vi "Init log file.vi"(8 "error in (no error)":errorcluster, 11 "Channel in":refnum<class "Channel.lvclass">) -> (0 "error out":errorcluster, 3 "Channel out":refnum<class "Channel.lvclass">)   [LabVIEW 2018, in "Channel.lvclass"]
uses:
  Channel.lvclass
  Error log/Error log.lvclass
  C:/Users/Denis/Desktop/S4ACS/SPARC4_ACS/Log File/Log File.lvclass
  Keywords Log File/Keywords Log File.lvclass
  Channel.lvclass/Channel.ctl
  Log File/Log File.lvclass/Log File.ctl
  Log File/Log File.lvclass
panel:
  in  "Keywords Log File.lvclass":refnum<class "Keywords Log File.lvclass">
  in  "Error log.lvclass":refnum<class "Error log.lvclass">
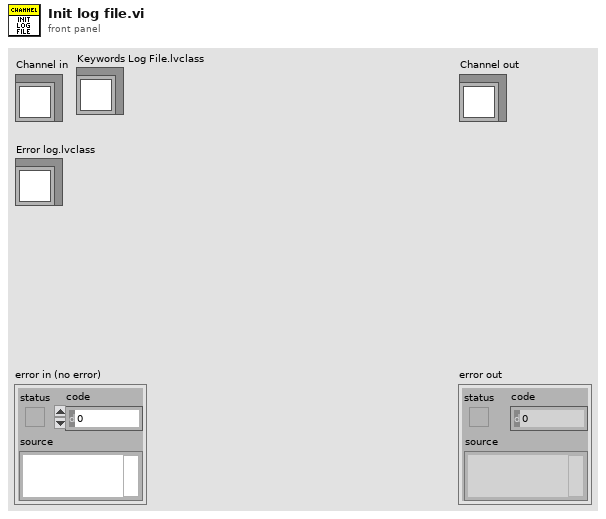
[diagram p1: front panel]
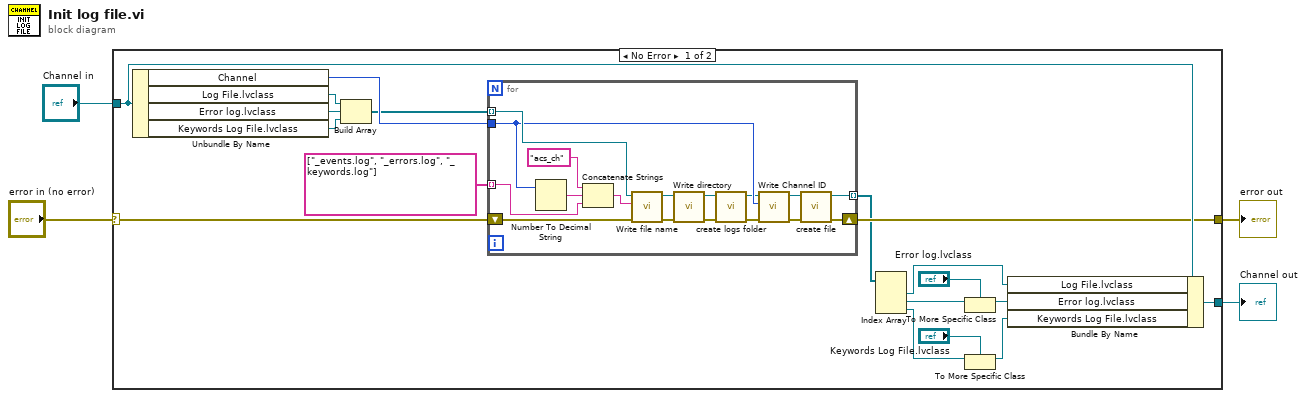
[diagram p0: block diagram]
diagram:
  n1 = case shown="No Error" "error in (no error)" {
    selector: "error in (no error)" -> [w22 w41]
    tunnel: [w20 w41] -> w3
    tunnel: [w19 w40] -> w1
    tunnel: "Channel in" -> [w21 w40]
    frame No Error {
      n2 = Unbundle By Name(w21) -> ("Channel"=w18:u8, "Log File.lvclass"=w17:refnum<class "Log File.lvclass">, "Error log.lvclass"=w16:refnum<class "Error log.lvclass">, "Keywords Log File.lvclass"=w15:refnum<class "Keywords Log File.lvclass">)
      n3 = Build Array(w17, w16, w15) -> (w14:refnum<class "Log File.lvclass">[])
      n4 = for {
        tunnel: w18 -> [w30]
        shift-right: [w34] -> w20
        shift-left: w22 -> [w35]
        tunnel: w14 -> [w33] mode=indexing
        tunnel: [w32] -> w13 mode=indexing
        tunnel: string[] ["_events.log", "_errors.log", "_keywords.log"] -> [w28] mode=indexing
        n5 = Number To Decimal String(number=w30) -> (decimal integer string=w29:string)  [unwired: 1 in]
        n6 = Concatenate Strings("acs_ch" ("file name"), w29, w28) -> (w27:string)
        n7 = call "Write file name.vi"("error in (no error)"=w35, "file name"=w27, "Log File in"=w33) -> ("error out"=w38:errorcluster, "Log File out"=w39:refnum<class "Log File.lvclass">)  [unwired: 7 in]
        n8 = call "Write directory.vi"("error in (no error)"=w38, "Log File in"=w39) -> ("error out"=w23:errorcluster, "Log File out"=w26:refnum<class "Log File.lvclass">)  [unwired: 8 in]
        n9 = call "create logs folder.vi"("error in (no error)"=w23, "Log File in"=w26) -> ("error out"=w24:errorcluster, "Log File out"=w25:refnum<class "Log File.lvclass">)  [unwired: 8 in]
        n10 = call "Write Channel ID.vi"("error in (no error)"=w24, "Channel ID"=w30, "Log File in"=w25) -> ("error out"=w37:errorcluster, "Log File out"=w36:refnum<class "Log File.lvclass">)  [unwired: 7 in]
        n11 = call "create file.vi"("error in (no error)"=w37, "Log File in"=w36) -> ("error out"=w34:errorcluster, "Log File out"=w32:refnum<class "Log File.lvclass">)  [unwired: 8 in]
      }
      n12 = Index Array(array=w13) -> (element #1=w12:refnum<class "Log File.lvclass">, element #2=w11:refnum<class "Log File.lvclass">, element #3=w8:refnum<class "Log File.lvclass">)  [unwired: 3 in]
      n13 = To More Specific Class(target class="Error log.lvclass", reference=w11) -> (specific class reference=w10:refnum<class "Error log.lvclass">)  [unwired: 1 in, 1 out]
      n14 = To More Specific Class(target class="Keywords Log File.lvclass", reference=w8) -> (specific class reference=w7:refnum<class "Keywords Log File.lvclass">)  [unwired: 1 in, 1 out]
      n15 = Bundle By Name(cluster=w21, "Log File.lvclass"=w12, "Error log.lvclass"=w10, "Keywords Log File.lvclass"=w7) -> (w19:refnum<class "Channel.lvclass">)
    }
    frame Error {
    }
  }
  "error out" <- w3
  "Channel out" <- w1
